vi "Get_Climber_Switches.vi"() -> (3 "climber_sensor_readings":T1)   [LabVIEW 2012]
uses:
  climber_sensor_readings.ctl
  <vilib>/Rock Robotics/WPI/CAN/Jaguar/SubVIs/WPI_CANJaguar_StatusSelect.ctl
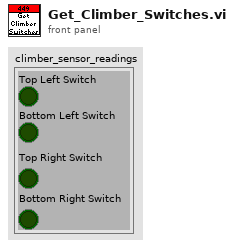
[diagram p1: front panel]
types:
  T1 = typedef "climber_sensor_readings.ctl" = cluster{"Top Left Switch":bool, "Bottom Left Switch":bool, "Top Right Switch":bool, "Bottom Right Switch":bool}
  T2 = typedef "WPI_CANJaguar_StatusSelect.ctl" = enum16{"Output Percent VBus", "Output Voltage", "Bus Voltage", "Current", "Temperature", "Position", "Speed", "Limit Switches", "Faults", "Fault Counters", "Power Cycle"}
  T3 = typedef "WPI_MotorControlDeviceRef.ctl" = cluster{"DeviceStatus":errorcluster, "Type":enum16{"PWM", "CAN"}, "PWM":cluster{"Digital Module":T4, "PWM Channel":T5, "DeadBand":T6}, "CAN":cluster{"Device Number":u8, "Control Mode":T7, "Semaphore":T8, "Max Vout":dbl}, "Invert":bool, "TransformRef":T9, "InvTransformRef":T9}
  T4 = typedef "FPGA_TypedefDigitalModule.ctl" = enum16{"Digital Module 1", "Digital Module 2"}
  T5 = typedef "FPGA_DIOPWMChannel.ctl" = enum8{"PWM 1", "PWM 2", "PWM 3", "PWM 4", "PWM 5", "PWM 6", "PWM 7", "PWM 8", "PWM 9", "PWM 10", "Invalid"}
  T6 = typedef "WPI_PWMDeadband.ctl" = cluster{"Name":string, "maxPositivePwm":i32, "minPositivePwm":i32, "centerPwm":i32, "maxNegativePwm":i32, "minNegativePwm":i32, "angularRange":u16}
  T7 = typedef "WPI_CANJaguar_ControlMode.ctl" = enum8{"Percent VBus", "Current", "Speed", "Position", "Voltage"}
  T8 = typedef "Semaphore RefNum" = refnum<k1>
  T9 = typedef "WPI_PWMTransform_ConPane.ctl" = refnum<vi>
  T10 = typedef "WPI_CANJaguar_Status.ctl" = cluster{"Output Percent VBus":dbl, "Output Voltage":dbl, "Bus Voltage":dbl, "Current":dbl, "Temperature":dbl, "Position":dbl, "Speed":dbl, "Limits":cluster{"Forward Limit":bool, "Reverse Limit":bool, "Forward Soft Limit":bool, "Reverse Soft Limit":bool, "Sticky Forward Limit":bool, "Sticky Reverse Limit":bool, "Sticky Forward Soft Limit":bool, "Sticky Reverse Soft Limit":bool}, "Faults":cluster{"Current Fault":bool, "Temperature Fault":bool, "Bus Voltage Fault":bool, "Gate Driver Fault":bool, "Comm Fault":bool}, "Fault Counters":cluster{"Current Faults":u8, "Temperature Faults":u8, "Bus Voltage Faults":u8, "Gate Driver Faults":u8, "Comm Faults":u8, "CAN Status":u8, "CAN RX Errors":u8, "CAN TX Errors":u8}, "Power Cycle":bool}
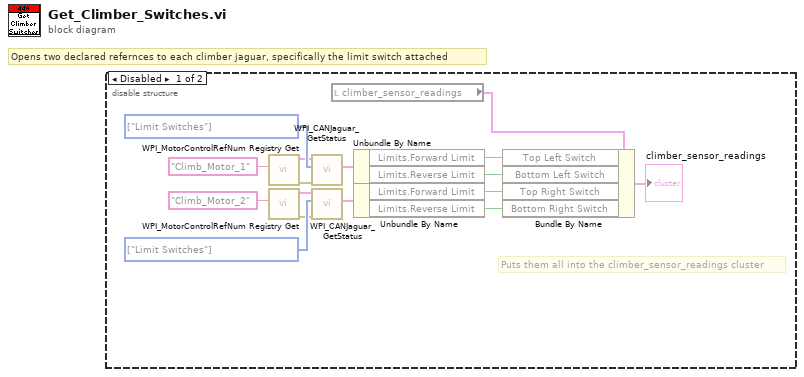
[diagram p0: block diagram]
diagram:
  # "Opens two declared refernces to each climber jaguar, specifically the limit switch attached"
  n1 = disable-structure shown="Disabled" {
    frame Disabled {
      w9 = T2[] [enum."Limit Switches"] items=["Output Percent VBus", "Output Voltage", "Bus Voltage", "Current", "Temperature", "Position", "Speed", "Limit Switches", "Faults", "Fault Counters", "Power Cycle"] ("Status Select")
      w14 = T2[] [enum."Limit Switches"] items=["Output Percent VBus", "Output Voltage", "Bus Voltage", "Current", "Temperature", "Position", "Speed", "Limit Switches", "Faults", "Fault Counters", "Power Cycle"] ("Status Select")
      # "Puts them all into the climber_sensor_readings cluster"
      n2 = call <vilib>:"WPI_MotorControlRefNum Registry Get.vi"("refnum name"="Climb_Motor_1") -> ("error out"=w10:errorcluster, "MotorControlDevRef"=w11:T3)  [unwired: 9 in]
      n3 = call <vilib>:"WPI_MotorControlRefNum Registry Get.vi"("refnum name"="Climb_Motor_2") -> ("error out"=w5:errorcluster, "MotorControlDevRef"=w6:T3)  [unwired: 9 in]
      n4 = call <vilib>:"WPI_CANJaguar_GetStatus.vi"("error in (no error)"=w10, "Status Select"=w14, "CAN Jaguar Ref"=w11) -> ("Status"=w13:T10)  [unwired: 6 in, 2 out]
      n5 = call <vilib>:"WPI_CANJaguar_GetStatus.vi"("error in (no error)"=w5, "Status Select"=w9, "CAN Jaguar Ref"=w6) -> ("Status"=w8:T10)  [unwired: 6 in, 2 out]
      n6 = local read "climber_sensor_readings"() -> (w15:T1)
      n7 = Unbundle By Name(w13) -> ("Limits.Forward Limit"=w4:bool, "Limits.Reverse Limit"=w3:bool)
      n8 = Unbundle By Name(w8) -> ("Limits.Forward Limit"=w2:bool, "Limits.Reverse Limit"=w1:bool)
      n9 = Bundle By Name(cluster=w15, "Top Left Switch"=w4, "Bottom Left Switch"=w3, "Top Right Switch"=w2, "Bottom Right Switch"=w1) -> (→"climber_sensor_readings":T1)
    }
    frame Enabled {
    }
  }
